vi "Array of Arrays to 2D Array.vi"(8 "error in (no error)":errorcluster, 11 "Variant in":variant) -> (0 "error out":errorcluster, 2 "Array Present?":bool, 3 "Variant out":variant)   [LabVIEW 2015]
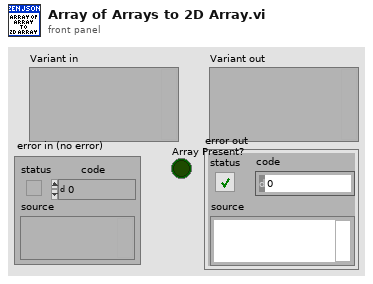
[diagram p1: front panel]
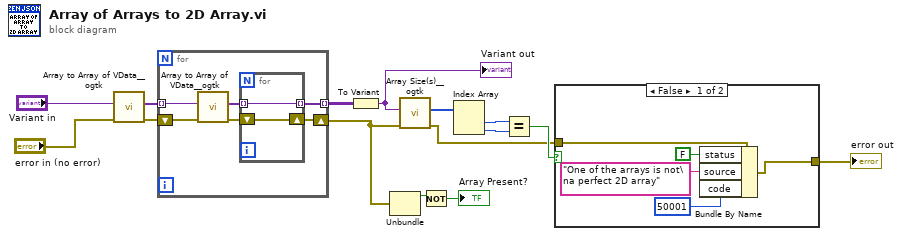
[diagram p0: block diagram]
diagram:
  n1 = call <userlib>:"Array to Array of VData__ogtk.vi"("error in (no error)"="error in (no error)", "MultiD Array"="Variant in") -> ("error out"=w11:errorcluster, "1D Array of Variants"=w14:variant[])  [unwired: 8 in]
  n2 = for {
    tunnel: w14 -> [w21] mode=indexing
    tunnel: [w19] -> w15 mode=indexing
    shift-right: [w17] -> w3
    shift-left: w11 -> [w18]
    n3 = call <userlib>:"Array to Array of VData__ogtk.vi"("error in (no error)"=w18, "MultiD Array"=w21) -> ("error out"=w16:errorcluster, "1D Array of Variants"=w20:variant[])  [unwired: 8 in]
    n4 = for {
      tunnel: w20 -> [w23] mode=indexing
      tunnel: [w23] -> w19 mode=indexing
      shift-right: [w22] -> w17
      shift-left: w16 -> [w22]
    }
  }
  n5 = To Variant(anything=w15) -> (Variant=w1:variant)
  "Variant out" <- w1
  n6 = Unbundle(w3) -> ("status"=w10:bool)  [unwired: 2 out]
  n7 = call <userlib>:"Array Size(s)__ogtk.vi"("error in (no error)"=w3, "Array"=w1) -> ("error out"=w2:errorcluster, "Size(s)"=w8:u32[])  [unwired: 7 in, 1 out]
  n8 = Not(x=w10) -> (.not. x?=→"Array Present?":bool)
  n9 = Index Array(array=w8) -> (element #1=w7:u32, element #2=w6:u32)  [unwired: 2 in]
  n10 = Equal?(x=w7, y=w6) -> (x = y?=w5:bool)
  n11 = case shown="False" w5 {
    tunnel: w2 -> [w28 w29]
    tunnel: [w26 w29] -> w4
    frame False {
      n12 = Bundle By Name(cluster=w28, "status"=FALSE, "source"="One of the arrays is not\na perfect 2D array", "code"=50001) -> (w26:errorcluster)
    }
    frame True {
    }
  }
  "error out" <- w4
